vi "Documentation.vi"   [LabVIEW 2019, in "Instrument.AFM_DLog.lvclass"]
uses:
  Instrument.AFM_DLog.lvclass
  d6248588-9140-4ff5-86c8-21cd21a7458c.vi
  7f72b22a-d2f9-4e7f-a221-6a14f9895fe8.vi
  7f72b22a-d2f9-4e7f-a221-6a14f9895fe8.vi/42f86bcf-068c-4498-966d-034f8f180634.vi
  7f72b22a-d2f9-4e7f-a221-6a14f9895fe8.vi/bd09be8a-821b-4106-aeb3-ddc481226dfb.vi
  <vilib>/Utility/Data Type/Get Type Information.vi
  <vilib>/Utility/Data Type/Get Numeric Information.vi
  <userlib>/_OpenG.lib/lvdata/lvdata.llb/Unwrap VVariant__ogtk.vi
  <vilib>/JDP Science/JSONtext/JSON text to Variant.vi
  <userlib>/LevyLab/Instrument Framework/Instrument/Instrument.lvclass
  <vilib>/JKI/JKI SMO/SMO/SMO.lvclass
  Typedefs/Instrument.AFM_DLog.PublicCommands--Enum.ctl
  Typedefs/Instrument.AFM_DLog.getAll--Cluster.ctl
  Typedefs/Instrument.AFM_DLog.Configuration--Cluster.ctl
  Typedefs/Instrument.AFM_DLog.ProtectedCommands--Enum.ctl
  <vilib>/JDP Science/JSONtext/LVClass Serializer/JSONtext LVClass Serializer.lvclass
  <userlib>/LevyLab/Instrument Framework/Instrument UI/Instrument UI.lvclass
  <userlib>/LevyLab/Instrument Framework/Instrument Types/Amplifier/Instrument.Amplifier.lvclass
  <userlib>/LevyLab/Instrument Framework/Instrument Types/CBridge/Instrument.CBridge.lvclass
  <userlib>/LevyLab/Instrument Framework/Instrument Types/Cryostat/Instrument.Cryostat.lvclass
  <userlib>/LevyLab/Instrument Framework/Instrument Types/Delay Line/Instrument.DelayLine.lvclass
  <userlib>/LevyLab/Instrument Framework/Instrument Types/Lockin/Instrument.LockinAPI.lvclass
  <userlib>/LevyLab/Instrument Framework/Instrument Types/Strain/Instrument.Strain.lvclass
  <userlib>/LevyLab/Instrument Framework/Instrument Types/VNA/Instrument.VNA.lvclass
  <userlib>/LevyLab/Instrument Framework/Instrument Types/SCPI/Instrument.SCPI.lvclass
  <userlib>/LevyLab/Instrument Framework/Instrument Types/SignalGenerator/Instrument.SignalGenerator.lvclass
  <userlib>/LevyLab/Instrument Framework/Instrument Types/VSource/Instrument.VSource.lvclass
  Instrument UI.AFM_DLog/Instrument UI.AFM_DLog.UI--Cluster.ctl
  <vilib>/JKI/JKI SMO/SMO.UI/SMO.UI.lvclass
  C:/Program Files (x86)/National Instruments/LabVIEW 2019/user.lib/LevyLab/Instrument Framework/Instrument/Instrument.lvclass
  C:/Program Files (x86)/National Instruments/LabVIEW 2019/vi.lib/JKI/JKI SMO/SMO/SMO.lvclass
  <userlib>/LevyLab/Instrument Framework/Instrument/Typedefs/Instrument.ProtectedCommands--Enum.ctl
  <userlib>/LevyLab/Instrument Framework/Instrument/Typedefs/Instrument.Commands--Enum.ctl
types:
  T1 = typedef "Instrument.AFM_DLog.lvclass/Instrument.AFM_DLog.Configuration--Cluster.ctl" = cluster{"Example Setting 1":dbl, "Example Setting 2":dbl, "Example Setting 3":string}
  T2 = typedef "Instrument.AFM_DLog.lvclass/Instrument.AFM_DLog.getAll--Cluster.ctl" = cluster{"Name":string, "X":dbl, "Y":dbl, "Speed":dbl, "Voltage":dbl, "Set Resistance":string, "Move Setpoint":dbl, "Amplifier":dbl, "Writing Setpoint":dbl, "Interpolation":dbl}
  T3 = typedef "Instrument.AFM_DLog.lvclass/Instrument.AFM_DLog.ProtectedCommands--Enum.ctl" = enum16{"doProtected"}
  T4 = typedef "Instrument.AFM_DLog.lvclass/Instrument.AFM_DLog.PublicCommands--Enum.ctl" = enum16{"doSomething"}
  T5 = typedef "Instrument.lvlib/Instrument.lvclass/Instrument.Commands--Enum.ctl" = enum16{"ACK", "HELP", "IDN", "getAll", "getAllData"}
  T6 = typedef "Instrument.lvlib/Instrument.lvclass/Instrument.ProtectedCommands--Enum.ctl" = enum16{"setConfiguration", "setIDN", "setAll", "setAllData"}
  T7 = typedef "Instrument UI.AFM_DLog.lvclass/Instrument UI.AFM_DLog.UI--Cluster.ctl" = cluster{"Parameter":dbl, "Parameter 2":string}
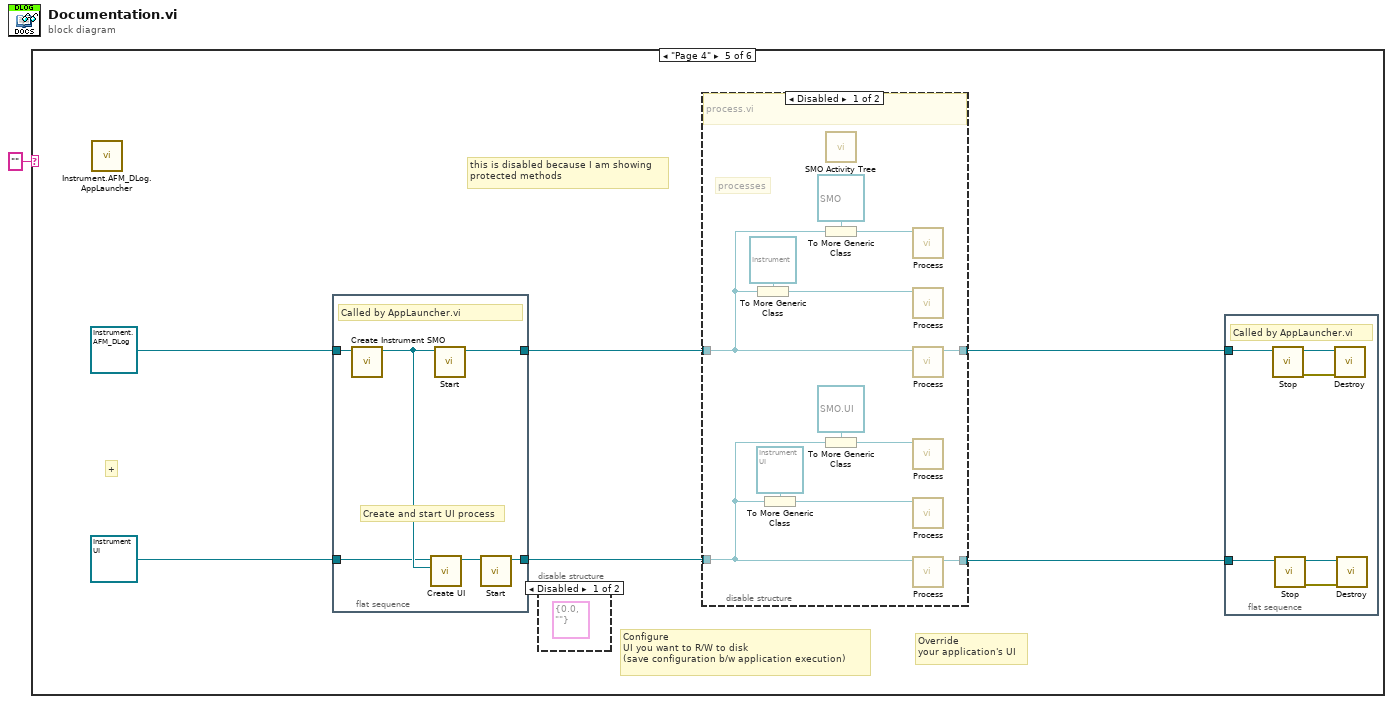
[diagram p0: block diagram]
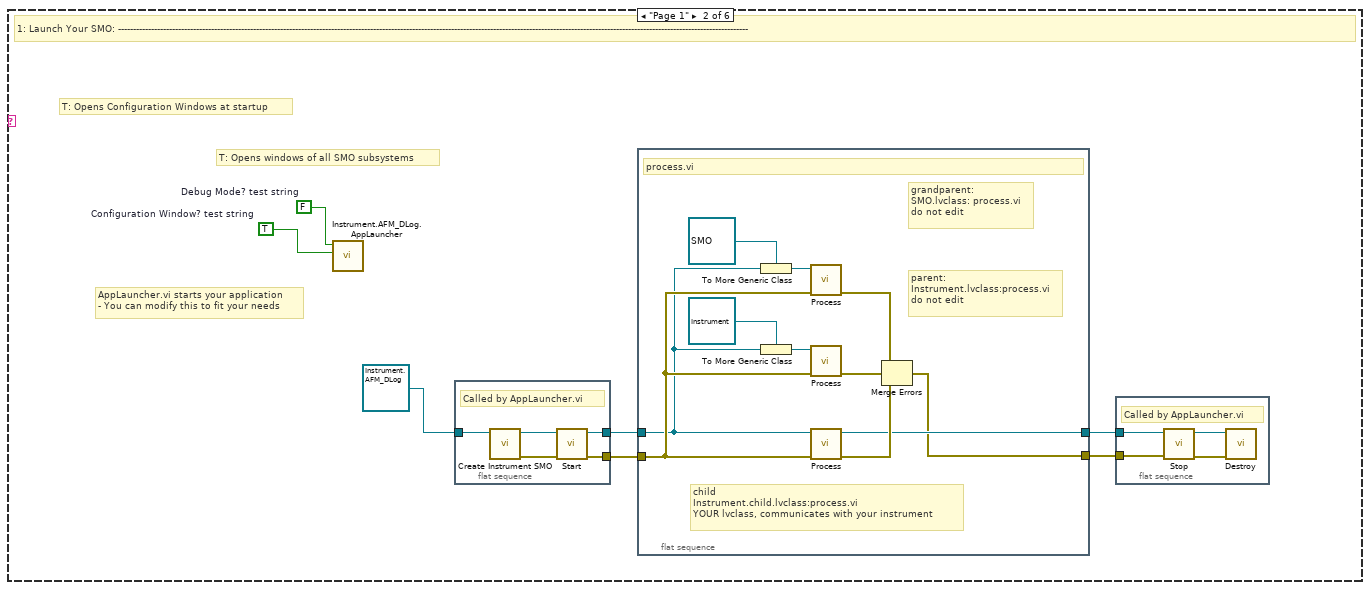
[diagram p3: hidden frame]
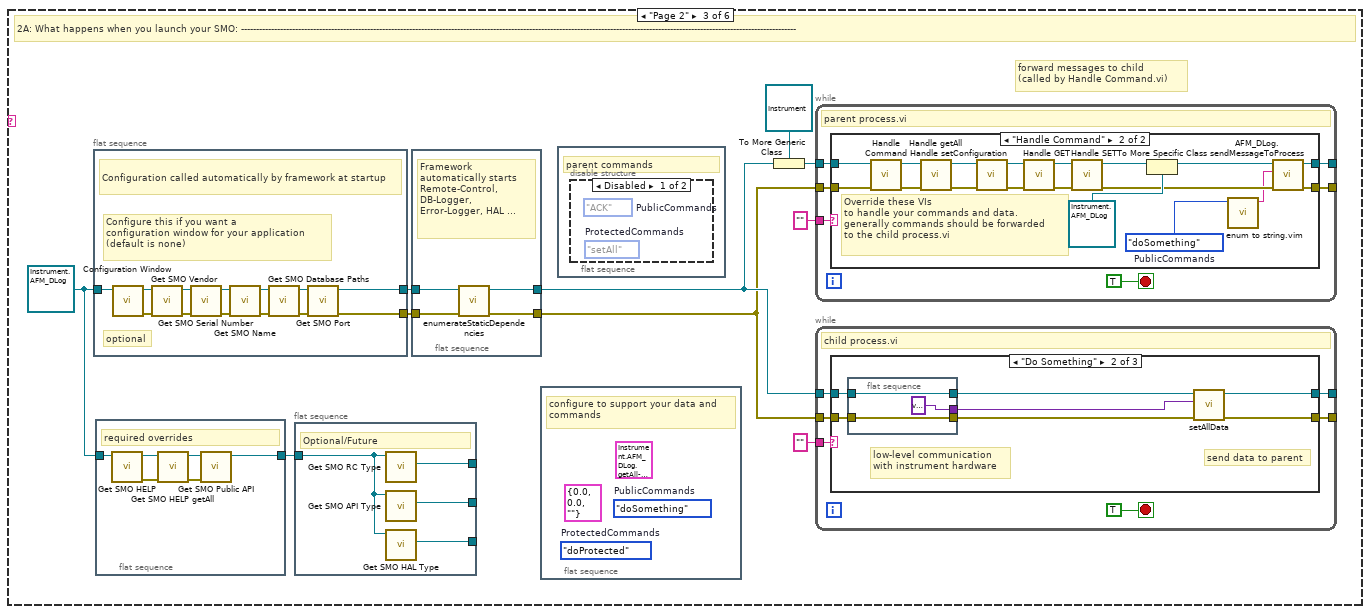
[diagram p4: hidden frame]
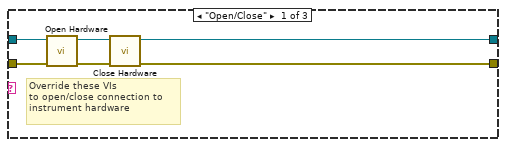
[diagram p6: hidden frame]
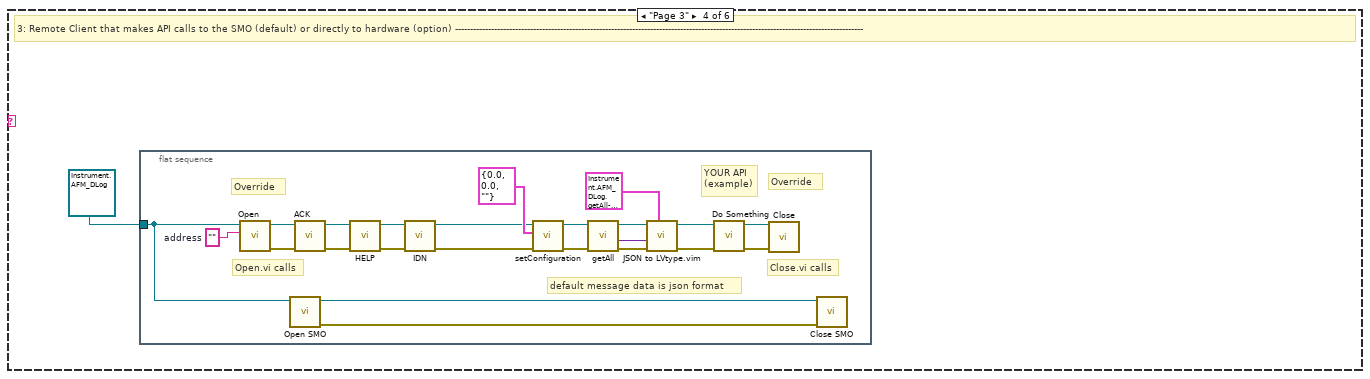
[diagram p9: hidden frame]
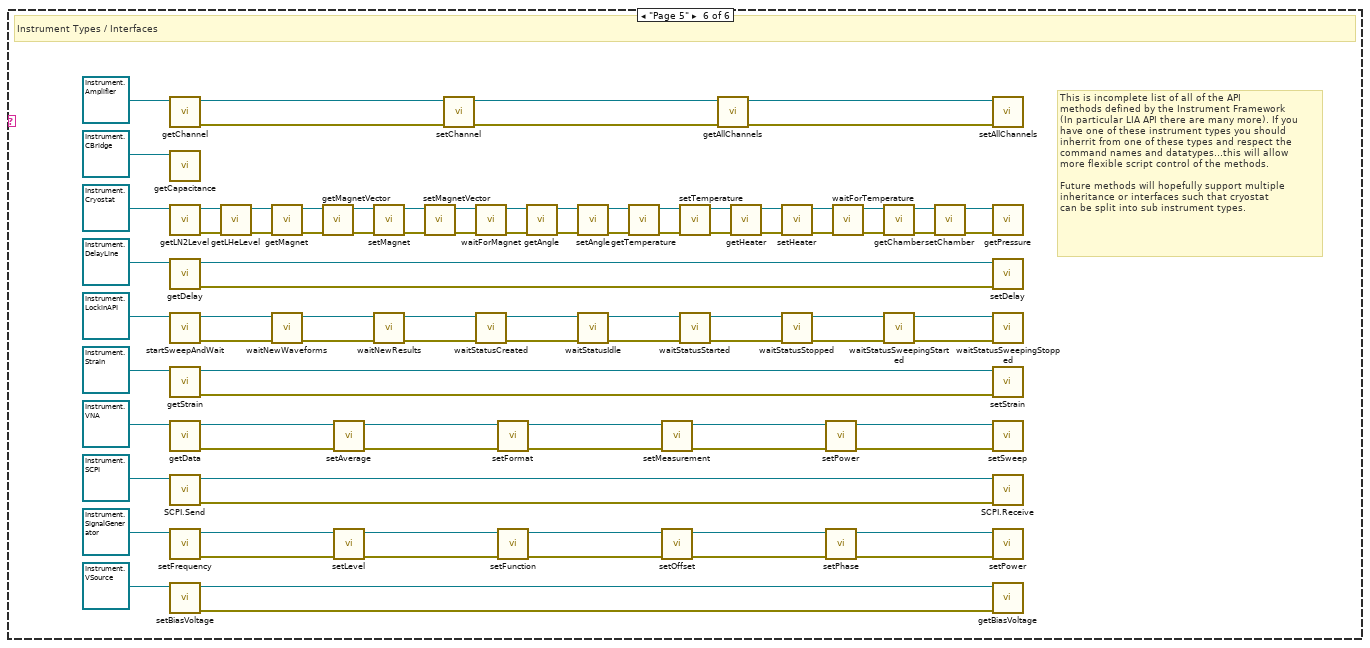
[diagram p12: hidden frame]
diagram:
  n1 = case shown="\"Page 4\"" "" {
    frame Default {
    }
    frame "Page 1" {
      w7 = TRUE  # Configuration Window? test string
      w8 = FALSE  # Debug Mode? test string
      # "AppLauncher.vi starts your application\n- You can modify this to fit your needs"
      # "T: Opens windows of all SMO subsystems"
      # "T: Opens Configuration Windows at startup"
      # "1: Launch Your SMO: ------------------------------------------------------------------------------------------------------------------------------------------------------------------------------------------------------------------"
      n2 = call "Instrument.AFM_DLog.AppLauncher.vi"("Config Window"=w7, "Debug Mode"=w8) -> ()  [unwired: 9 in, 1 out]
      n3 = flat-sequence {
        tunnel: [w26] -> w3
        tunnel: [w25] -> w5
        tunnel: refnum<class "Instrument.AFM_DLog.lvclass"> refnum ("Instrument.Template.lvclass") -> [w24]
        frame #0 {
          # "Called by AppLauncher.vi"
          n4 = call <userlib>:"Create Instrument SMO.vi"("Instrument in"=w24) -> ("error out"=w27:errorcluster, "Instrument out"=w28:refnum<class "Instrument.AFM_DLog.lvclass">)  [unwired: 9 in]
          n5 = call <vilib>:"Start.vi"("error in (no error)"=w27, "SMO"=w28) -> ("error out"=w25:errorcluster, "SMO out"=w26:refnum<class "Instrument.AFM_DLog.lvclass">)  [unwired: 8 in]
        }
      }
      n6 = flat-sequence {
        tunnel: [w10] -> w6
        tunnel: w5 -> [w18]
        tunnel: [w13] -> w4
        tunnel: w3 -> [w12]
        frame #0 {
          # "child\nInstrument.child.lvclass:process.vi\nYOUR lvclass, communicates with your instrument"
          # "grandparent:\nSMO.lvclass: process.vi\ndo not edit"
          # "parent:\nInstrument.lvclass:process.vi\ndo not edit"
          # "process.vi"
          n7 = To More Generic Class(target class=refnum<class "SMO.lvclass"> refnum ("SMO"), reference=w12) -> (generic class reference=w19:refnum<class "SMO.lvclass">)
          n8 = To More Generic Class(target class=refnum<class "Instrument.lvclass"> refnum ("Instrument"), reference=w12) -> (generic class reference=w17:refnum<class "Instrument.lvclass">)
          n9 = call-dynamic "Process.vi"("error in"=w18, "SMO"=w19) -> ("error out"=w14:errorcluster)  [unwired: 8 in, 1 out]
          n10 = call-dynamic "Process.vi"("error in"=w18, "Instrument"=w17) -> ("error out"=w16:errorcluster)  [unwired: 8 in, 1 out]
          n11 = call-dynamic "Process.vi"("error in"=w18, "Instrument.AFM_DLog in"=w12) -> ("error out"=w15:errorcluster, "Instrument.AFM_DLog out"=w13:refnum<class "Instrument.AFM_DLog.lvclass">)  [unwired: 8 in]
          n12 = Merge Errors(w14, w16, w15) -> (w10:errorcluster)
        }
      }
      n13 = flat-sequence {
        tunnel: w4 -> [w21]
        tunnel: w6 -> [w20]
        frame #0 {
          # "Called by AppLauncher.vi"
          n14 = call <vilib>:"Stop.vi"("error in (no error)"=w20, "SMO"=w21) -> ("error out"=w23:errorcluster, "SMO out"=w22:refnum<class "Instrument.AFM_DLog.lvclass">)  [unwired: 8 in]
          n15 = call <vilib>:"Destroy.vi"("error in (no error)"=w23, "SMO"=w22) -> ()  [unwired: 9 in, 1 out]
        }
      }
    }
    frame "Page 2" {
      w32 = refnum<class "Instrument.AFM_DLog.lvclass"> refnum ("Instrument.Template.lvclass")
      # "forward messages to child\n(called by Handle Command.vi)"
      # "2A: What happens when you launch your SMO: -----------------------------------------------------------------------------------------------------------------------------------------------------------------------------------------"
      n16 = flat-sequence {
        tunnel: w32 -> [w59]
        tunnel: [w49] -> w33
        tunnel: [w50] -> w34
        frame #0 {
          # "optional"
          # "Configure this if you want a\nconfiguration window for your application\n(default is none)"
          # "Configuration called automatically by framework at startup"
          n17 = call-dynamic "Configuration Window.vi"("Example Instrument in"=w59) -> ("error out"=w61:errorcluster, "Example Instrument out"=w60:refnum<class "Instrument.AFM_DLog.lvclass">)  [unwired: 9 in]
          n18 = call-dynamic "Get SMO Vendor.vi"("error in (no error)"=w61, "Instrument.AFM_DLog in"=w60) -> ("error out"=w51:errorcluster, "Instrument.AFM_DLog out"=w56:refnum<class "Instrument.AFM_DLog.lvclass">)  [unwired: 7 in, 1 out]
          n19 = call-dynamic "Get SMO Serial Number.vi"("error in (no error)"=w51, "Instrument.AFM_DLog in"=w56) -> ("error out"=w52:errorcluster, "Instrument.AFM_DLog out"=w55:refnum<class "Instrument.AFM_DLog.lvclass">)  [unwired: 7 in, 1 out]
          n20 = call-dynamic "Get SMO Name.vi"("error in (no error)"=w52, "Instrument.AFM_DLog in"=w55) -> ("error out"=w53:errorcluster, "Instrument.AFM_DLog out"=w54:refnum<class "Instrument.AFM_DLog.lvclass">)  [unwired: 7 in, 1 out]
          n21 = call-dynamic "Get SMO Database Paths.vi"("error in (no error)"=w53, "Instrument.AFM_DLog in"=w54) -> ("error out"=w57:errorcluster, "Instrument.AFM_DLog out"=w58:refnum<class "Instrument.AFM_DLog.lvclass">)  [unwired: 7 in, 1 out]
          n22 = call-dynamic "Get SMO Port.vi"("error in (no error)"=w57, "Instrument.AFM_DLog in"=w58) -> ("error out"=w49:errorcluster, "Instrument.AFM_DLog out"=w50:refnum<class "Instrument.AFM_DLog.lvclass">)  [unwired: 7 in, 1 out]
        }
      }
      n23 = flat-sequence {
        tunnel: w32 -> [w40]
        tunnel: [w39] -> w31
        frame #0 {
          # "required overrides"
          n24 = call-dynamic "Get SMO HELP.vi"("Instrument.AFM_DLog in"=w40) -> ("error out"=w44:errorcluster, "Instrument.AFM_DLog out"=w43:refnum<class "Instrument.AFM_DLog.lvclass">)  [unwired: 8 in, 1 out]
          n25 = call-dynamic "Get SMO HELP getAll.vi"("error in (no error)"=w44, "Instrument.AFM_DLog in"=w43) -> ("error out"=w41:errorcluster, "Instrument.AFM_DLog out"=w42:refnum<class "Instrument.AFM_DLog.lvclass">)  [unwired: 7 in, 1 out]
          n26 = call-dynamic "Get SMO Public API.vi"("error in (no error)"=w41, "Instrument.AFM_DLog in"=w42) -> ("Instrument.AFM_DLog out"=w39:refnum<class "Instrument.AFM_DLog.lvclass">)  [unwired: 7 in, 2 out]
        }
      }
      n27 = flat-sequence {
        tunnel: w31 -> [w65]
        tunnel: [w64] -> _
        tunnel: [w63] -> _
        tunnel: [w62] -> _
        frame #0 {
          # "Optional/Future"
          n28 = call-dynamic "Get SMO RC Type.vi"("Instrument in"=w65) -> ("RemoteControl"=w64:refnum<class "RemoteControl.lvclass">)  [unwired: 8 in, 2 out]
          n29 = call-dynamic "Get SMO API Type.vi"("Instrument in"=w65) -> ("API"=w63:refnum<class "API.lvclass">)  [unwired: 8 in, 2 out]
          n30 = call-dynamic "Get SMO HAL Type.vi"("Instrument in"=w65) -> ("Dependencies.HAL"=w62:refnum<class "HAL.lvclass">)  [unwired: 8 in, 2 out]
        }
      }
      n31 = flat-sequence {
        tunnel: w34 -> [w48]
        tunnel: w33 -> [w47]
        tunnel: [w46] -> w30
        tunnel: [w45] -> w29
        frame #0 {
          # "Framework automatically starts\nRemote-Control, DB-Logger, Error-Logger, HAL ..."
          n32 = call-dynamic "enumerateStaticDependencies.vi"("error in (no error)"=w47, "Instrument"=w48) -> ("error out"=w45:errorcluster, "Instrument out"=w46:refnum<class "Instrument.AFM_DLog.lvclass">)  [unwired: 7 in, 1 out]
        }
      }
      n33 = flat-sequence {
        frame #0 {
          (unwired) Instrument.AFM_DLog.ProtectedCommands--Enum."doProtected"  # ProtectedCommands
          (unwired) T1 {"Example Setting 1"=0.0, "Example Setting 2"=0.0, "Example Setting 3"=""} ("Configuration")
          (unwired) T2 {"Name"="", "X"=0.0, "Y"=0.0, "Speed"=0.0, "Voltage"=0.0, "Set Resistance"="", "Move Setpoint"=0.0, "Amplifier"=0.0, "Writing Setpoint"=0.0, "Interpolation"=0.0} ("getAll")
          (unwired) Instrument.AFM_DLog.PublicCommands--Enum."doSomething"  # PublicCommands
          # "configure to support your data and commands"
        }
      }
      n34 = flat-sequence {
        frame #0 {
          # "parent commands"
          n35 = disable-structure shown="Disabled" {
            frame Disabled {
              (unwired) Instrument.Commands--Enum."ACK"  # PublicCommands
              (unwired) Instrument.ProtectedCommands--Enum."setAll"  # ProtectedCommands
            }
            frame Enabled {
            }
          }
        }
      }
      n36 = To More Generic Class(target class=refnum<class "Instrument.lvclass"> refnum ("Instrument"), reference=w30) -> (generic class reference=w35:refnum<class "Instrument.lvclass">)
      n37 = while {
        tunnel: "" -> [w95]
        tunnel: w35 -> [w93]
        tunnel: [w92] -> _
        tunnel: w29 -> [w91]
        tunnel: [w90] -> _
        stop <- TRUE stop-if-true
        # "parent process.vi"
        n38 = case shown="\"Handle Command\"" w95 {
          tunnel: w93 -> [w97 w115]
          tunnel: [w97 w109] -> w92
          tunnel: w91 -> [w96 w114]
          tunnel: [w96 w108] -> w90
          frame Default {
          }
          frame "Handle Command" {
            w99 = Instrument.AFM_DLog.PublicCommands--Enum."doSomething"  # PublicCommands
            # "Override these VIs\nto handle your commands and data.\ngenerally commands should be forwarded\nto the child process.vi"
            n39 = call-dynamic "Handle Command.vi"("error in (no error)"=w114, "Instrument in"=w115) -> ("error out"=w110:errorcluster, "Instrument out"=w113:refnum<class "Instrument.lvclass">)  [unwired: 6 in, 2 out]
            n40 = call-dynamic "Handle getAll.vi"("error in (no error)"=w110, "Instrument in"=w113) -> ("error out"=w111:errorcluster, "Instrument out"=w112:refnum<class "Instrument.lvclass">)  [unwired: 7 in, 1 out]
            n41 = call-dynamic "Handle setConfiguration.vi"("error in (no error)"=w111, "Instrument in"=w112) -> ("error out"=w104:errorcluster, "Instrument out"=w105:refnum<class "Instrument.lvclass">)  [unwired: 8 in]
            n42 = call-dynamic "Handle GET.vi"("error in (no error)"=w104, "Instrument in"=w105) -> ("error out"=w102:errorcluster, "Instrument out"=w103:refnum<class "Instrument.lvclass">)  [unwired: 7 in, 1 out]
            n43 = call-dynamic "Handle SET.vi"("error in (no error)"=w102, "Instrument in"=w103) -> ("error out"=w100:errorcluster, "Instrument out"=w101:refnum<class "Instrument.lvclass">)  [unwired: 7 in, 1 out]
            n44 = To More Specific Class(target class=refnum<class "Instrument.AFM_DLog.lvclass"> refnum ("Instrument.Template.lvclass"), reference=w101) -> (specific class reference=w107:refnum<class "Instrument.AFM_DLog.lvclass">)  [unwired: 1 in, 1 out]
            n45 = call "enum to string.vim"("enum in"=w99) -> ("string out"=w98:string)  [unwired: 9 in, 1 out]
            n46 = call "AFM_DLog.sendMessageToProcess.vi"("error in (no error)"=w100, "Command"=w98, "Instrument.AFM_DLog in"=w107) -> ("error out"=w108:errorcluster, "Instrument.AFM_DLog out"=w109:refnum<class "Instrument.AFM_DLog.lvclass">)  [unwired: 7 in]
          }
        }
      }
      n47 = while {
        tunnel: "" -> [w71]
        tunnel: w30 -> [w69]
        tunnel: [w68] -> _
        tunnel: w29 -> [w67]
        tunnel: [w66] -> _
        stop <- TRUE stop-if-true
        # "child process.vi"
        n48 = case shown="\"Do Something\"" w71 {
          tunnel: w69 -> [w74 w83 w89]
          tunnel: [w73 w80 w89] -> w68
          tunnel: w67 -> [w77 w84 w88]
          tunnel: [w72 w79 w88] -> w66
          frame "Open/Close" {
            # "Override these VIs\nto open/close connection to\ninstrument hardware"
            n49 = call-dynamic "Open Hardware.vi"("error in (no error)"=w77, "Instrument in"=w74) -> ("error out"=w76:errorcluster, "Instrument out"=w75:refnum<class "Instrument.AFM_DLog.lvclass">)  [unwired: 8 in]
            n50 = call-dynamic "Close Hardware.vi"("error in (no error)"=w76, "Instrument in"=w75) -> ("error out"=w72:errorcluster, "Instrument out"=w73:refnum<class "Instrument.AFM_DLog.lvclass">)  [unwired: 8 in]
          }
          frame "Do Something" {
            # "low-level communication\nwith instrument hardware"
            # "send data to parent"
            n51 = flat-sequence {
              tunnel: w84 -> [w87]
              tunnel: [w87] -> w78
              tunnel: w83 -> [w86]
              tunnel: [w86] -> w81
              tunnel: [variant ("Data")] -> w82
              frame #0 {
              }
            }
            n52 = call <userlib>:"setAllData.vi"("error in (no error)"=w78, "AllData"=w82, "Instrument in"=w81) -> ("error out"=w79:errorcluster, "Instrument out"=w80:refnum<class "Instrument.AFM_DLog.lvclass">)  [unwired: 7 in]
          }
          frame Default {
          }
        }
      }
    }
    frame "Page 3" {
      # "3: Remote Client that makes API calls to the SMO (default) or directly to hardware (option) ----------------------------------------------------------------------------------------------------------------------------------------"
      n53 = flat-sequence {
        tunnel: refnum<class "Instrument.AFM_DLog.lvclass"> refnum ("Instrument.Template.lvclass") -> [w126]
        frame #0 {
          w129 = ""  # address
          # "default message data is json format"
          # "Close.vi calls"
          # "Open.vi calls"
          # "YOUR API\n(example)"
          # "Override"
          # "Override"
          n54 = call-dynamic "Open.vi"("address"=w129, "Instrument.AFM_DLog in"=w126) -> ("error out"=w138:errorcluster, "Instrument.AFM_DLog out"=w137:refnum<class "Instrument.AFM_DLog.lvclass">)  [unwired: 8 in]
          n55 = call <userlib>:"Open SMO.vi"("Instrument in"=w126) -> ("error out"=w127:errorcluster, "Instrument out"=w128:refnum<class "Instrument.AFM_DLog.lvclass">)  [unwired: 9 in]
          n56 = call <userlib>:"ACK.vi"("error in (no error)"=w138, "Instrument in"=w137) -> ("error out"=w136:errorcluster, "Instrument out"=w135:refnum<class "Instrument.AFM_DLog.lvclass">)  [unwired: 7 in, 1 out]
          n57 = call <userlib>:"HELP.vi"("error in (no error)"=w136, "Instrument in"=w135) -> ("error out"=w119:errorcluster, "Instrument in"=w120:refnum<class "Instrument.AFM_DLog.lvclass">)  [unwired: 7 in, 1 out]
          n58 = call <userlib>:"IDN.vi"("error in (no error)"=w119, "Instrument in"=w120) -> ("error out"=w117:errorcluster, "Instrument in"=w118:refnum<class "Instrument.AFM_DLog.lvclass">)  [unwired: 7 in, 1 out]
          n59 = call <userlib>:"setConfiguration.vi"("error in (no error)"=w117, "Configuration"=T1 {"Example Setting 1"=0.0, "Example Setting 2"=0.0, "Example Setting 3"=""}, "Instrument in"=w118) -> ("error out"=w130:errorcluster, "Instrument out"=w131:refnum<class "Instrument.AFM_DLog.lvclass">)  [unwired: 7 in]
          n60 = call <userlib>:"getAll.vi"("error in (no error)"=w130, "Instrument in"=w131) -> ("error out"=w125:errorcluster, "getAll"=w121:variant, "Instrument out"=w122:refnum<class "Instrument.AFM_DLog.lvclass">)  [unwired: 7 in]
          n61 = call "JSON to LVtype.vim"("type"=T2 {"Name"="", "X"=0.0, "Y"=0.0, "Speed"=0.0, "Voltage"=0.0, "Set Resistance"="", "Move Setpoint"=0.0, "Amplifier"=0.0, "Writing Setpoint"=0.0, "Interpolation"=0.0} ("getAll"), "error in (no error)"=w125, "JSON Data in"=w121) -> ("error out"=w123:errorcluster)  [unwired: 7 in, 1 out]
          n62 = call-dynamic "Do Something.vi"("error in (no error)"=w123, "Instrument.AFM_DLog in"=w122) -> ("error out"=w133:errorcluster, "Instrument.AFM_DLog out"=w134:refnum<class "Instrument.AFM_DLog.lvclass">)  [unwired: 8 in]
          n63 = call-dynamic "Close.vi"("error in (no error)"=w133, "Instrument.AFM_DLog in"=w134) -> ()  [unwired: 8 in, 2 out]
          n64 = call <userlib>:"Close SMO.vi"("error in (no error)"=w127, "Instrument in"=w128) -> ()  [unwired: 8 in, 2 out]
        }
      }
    }
    frame "Page 4" {
      # "this is disabled because I am showing\nprotected methods"
      # "Configure\nUI you want to R/W to disk\n(save configuration b/w application execution)"
      # "Override\nyour application's UI"
      # "+"
      n65 = call "Instrument.AFM_DLog.AppLauncher.vi"() -> ()  [unwired: 11 in, 1 out]
      n66 = flat-sequence {
        tunnel: [w156] -> w142
        tunnel: refnum<class "Instrument.AFM_DLog.lvclass"> refnum ("Instrument.Template.lvclass") -> [w155]
        tunnel: refnum<class "Instrument UI.lvclass"> refnum ("Instrument UI.Template.lvclass") -> [w153]
        tunnel: [w151] -> w140
        frame #0 {
          # "Create and start UI process"
          # "Called by AppLauncher.vi"
          n67 = call <userlib>:"Create Instrument SMO.vi"("Instrument in"=w155) -> ("Instrument out"=w154:refnum<class "Instrument.AFM_DLog.lvclass">)  [unwired: 9 in, 1 out]
          n68 = call <userlib>:"Create UI.vi"("Instrument in"=w154, "Instrument UI"=w153) -> ("Instrument UI out"=w152:refnum<class "Instrument UI.lvclass">)  [unwired: 8 in, 1 out]
          n69 = call <vilib>:"Start.vi"("SMO"=w154) -> ("SMO out"=w156:refnum<class "Instrument.AFM_DLog.lvclass">)  [unwired: 9 in, 1 out]
          n70 = call <vilib>:"Start.vi"("SMO"=w152) -> ("SMO out"=w151:refnum<class "Instrument UI.lvclass">)  [unwired: 9 in, 1 out]
        }
      }
      n71 = disable-structure shown="Disabled" {
        frame Disabled {
          (unwired) T7 {"Parameter"=0.0, "Parameter 2"=""} ("UI")
        }
        frame Enabled {
        }
      }
      n72 = disable-structure shown="Disabled" {
        disable-tunnel: [w168 w170] -> w143
        disable-tunnel: w142 -> [w167 w170]
        disable-tunnel: w140 -> [w166 w169]
        disable-tunnel: [w165 w169] -> w139
        frame Disabled {
          # "processes"
          # "process.vi"
          n73 = To More Generic Class(target class=refnum<class "Instrument.lvclass"> refnum ("Instrument"), reference=w167) -> (generic class reference=w163:refnum<class "Instrument.lvclass">)
          n74 = To More Generic Class(target class=refnum<class "Instrument UI.lvclass"> refnum ("Instrument UI"), reference=w166) -> (generic class reference=w159:refnum<class "Instrument UI.lvclass">)
          n75 = call <vilib>:"SMO Activity Tree.vi"() -> ()  [unwired: 12 in]
          n76 = To More Generic Class(target class=refnum<class "SMO.lvclass"> refnum ("SMO"), reference=w167) -> (generic class reference=w164:refnum<class "SMO.lvclass">)
          n77 = To More Generic Class(target class=refnum<class "SMO.UI.lvclass"> refnum ("SMO.UI"), reference=w166) -> (generic class reference=w157:refnum<class "SMO.UI.lvclass">)
          n78 = call-dynamic "Process.vi"("SMO"=w164) -> ()  [unwired: 9 in, 2 out]
          n79 = call-dynamic "Process.vi"("Instrument"=w163) -> ()  [unwired: 9 in, 2 out]
          n80 = call-dynamic "Process.vi"("Instrument.AFM_DLog in"=w167) -> ("Instrument.AFM_DLog out"=w168:refnum<class "Instrument.AFM_DLog.lvclass">)  [unwired: 9 in, 1 out]
          n81 = call-dynamic "Process.vi"("SMO.UI"=w157) -> ()  [unwired: 9 in, 2 out]
          n82 = call-dynamic "Process.vi"("Instrument UI in"=w159) -> ()  [unwired: 9 in, 2 out]
          n83 = call-dynamic "Process.vi"("Instrument UI in"=w166) -> ("Instrument UI out"=w165:refnum<class "Instrument UI.lvclass">)  [unwired: 9 in, 1 out]
        }
        frame Enabled {
        }
      }
      n84 = flat-sequence {
        tunnel: w143 -> [w148]
        tunnel: w139 -> [w146]
        frame #0 {
          # "Called by AppLauncher.vi"
          n85 = call <vilib>:"Stop.vi"("SMO"=w148) -> ("error out"=w150:errorcluster, "SMO out"=w149:refnum<class "Instrument.AFM_DLog.lvclass">)  [unwired: 9 in]
          n86 = call <vilib>:"Stop.vi"("SMO"=w146) -> ("error out"=w147:errorcluster, "SMO out"=w145:refnum<class "Instrument UI.lvclass">)  [unwired: 9 in]
          n87 = call <vilib>:"Destroy.vi"("error in (no error)"=w150, "SMO"=w149) -> ()  [unwired: 9 in, 1 out]
          n88 = call <vilib>:"Destroy.vi"("error in (no error)"=w147, "SMO"=w145) -> ()  [unwired: 9 in, 1 out]
        }
      }
    }
    frame "Page 5" {
      # "This is incomplete list of all of the API\nmethods defined by the Instrument Framework\n(In particular LIA API there are many more). If you\nhave one of these instrument types you should\ninherrit from one of these types and respect the \ncommand names and datatypes...this will allow\nmore flexible script control of the methods.\n\nFuture methods will hopefully support multiple\ninheritance or interfaces such that cryostat\ncan be split into sub instrument types."
      # "Instrument Types / Interfaces"
      n89 = call-dynamic "getChannel.vi"("Instrument.Amplifier in"=refnum<class "Instrument.Amplifier.lvclass"> refnum ("Instrument.Amplifier.lvclass")) -> ("error out"=w251:errorcluster, "Instrument.Amplifier out"=w252:refnum<class "Instrument.Amplifier.lvclass">)  [unwired: 8 in, 1 out]
      n90 = call-dynamic "getCapacitance.vi"("Instrument.CBridge in"=refnum<class "Instrument.CBridge.lvclass"> refnum ("Instrument.CBridge.lvclass")) -> ()  [unwired: 8 in, 3 out]
      n91 = call-dynamic "getLN2Level.vi"("Instrument.Cryostat in"=refnum<class "Instrument.Cryostat.lvclass"> refnum ("Instrument.Cryostat.lvclass")) -> ("error out"=w245:errorcluster, "Instrument.Cryostat out"=w246:refnum<class "Instrument.Cryostat.lvclass">)  [unwired: 8 in, 1 out]
      n92 = call <userlib>:"getDelay.vi"("Instrument.DelayLine in"=refnum<class "Instrument.DelayLine.lvclass"> refnum ("Instrument.DelayLine.lvclass")) -> ("error out"=w213:errorcluster, "Instrument.DelayLine out"=w214:refnum<class "Instrument.DelayLine.lvclass">)  [unwired: 7 in, 2 out]
      n93 = call-dynamic "startSweepAndWait.vi"("Instrument.LockinAPI in"=refnum<class "Instrument.LockinAPI.lvclass"> refnum ("Instrument.LockinAPI.lvclass")) -> ("error out"=w211:errorcluster, "Instrument.LockinAPI out"=w212:refnum<class "Instrument.LockinAPI.lvclass">)  [unwired: 9 in]
      n94 = call-dynamic "getStrain.vi"("Instrument.Strain in"=refnum<class "Instrument.Strain.lvclass"> refnum ("Instrument.Strain.lvclass")) -> ("error out"=w195:errorcluster, "Instrument.Strain out"=w196:refnum<class "Instrument.Strain.lvclass">)  [unwired: 8 in, 1 out]
      n95 = call-dynamic "getData.vi"("Instrument.VSource in"=refnum<class "Instrument.VNA.lvclass"> refnum ("Instrument.VNA.lvclass")) -> ("error out"=w193:errorcluster, "Instrument.VSource out"=w194:refnum<class "Instrument.VNA.lvclass">)  [unwired: 8 in, 1 out]
      n96 = call-dynamic "SCPI.Send.vi"("Instrument.SCPI in"=refnum<class "Instrument.SCPI.lvclass"> refnum ("Instrument.SCPI.lvclass")) -> ("error out"=w183:errorcluster, "Instrument.SCPI out"=w184:refnum<class "Instrument.SCPI.lvclass">)  [unwired: 9 in]
      n97 = call-dynamic "setFrequency.vi"("Instrument.SignalGenerator in"=refnum<class "Instrument.SignalGenerator.lvclass"> refnum ("Instrument.SignalGenerator.lvclass")) -> ("error out"=w181:errorcluster, "Instrument.SignalGenerator out"=w182:refnum<class "Instrument.SignalGenerator.lvclass">)  [unwired: 9 in]
      n98 = call-dynamic "setBiasVoltage.vi"("Instrument.VSource in"=refnum<class "Instrument.VSource.lvclass"> refnum ("Instrument.VSource.lvclass")) -> ("error out"=w171:errorcluster, "Instrument.VSource out"=w172:refnum<class "Instrument.VSource.lvclass">)  [unwired: 9 in]
      n99 = call-dynamic "getLHeLevel.vi"("error in (no error)"=w245, "Instrument.Cryostat in"=w246) -> ("error out"=w243:errorcluster, "Instrument.Cryostat out"=w244:refnum<class "Instrument.Cryostat.lvclass">)  [unwired: 7 in, 1 out]
      n100 = call-dynamic "getMagnet.vi"("error in (no error)"=w243, "Instrument.Cryostat in"=w244) -> ("error out"=w241:errorcluster, "Instrument.Cryostat out"=w242:refnum<class "Instrument.Cryostat.lvclass">)  [unwired: 5 in, 3 out]
      n101 = call-dynamic "waitNewWaveforms.vi"("error in (no error)"=w211, "Instrument.LockinAPI in"=w212) -> ("error out"=w209:errorcluster, "Instrument.LockinAPI out"=w210:refnum<class "Instrument.LockinAPI.lvclass">)  [unwired: 7 in, 1 out]
      n102 = call-dynamic "getMagnetVector.vi"("error in (no error)"=w241, "Instrument.Cryostat in"=w242) -> ("error out"=w239:errorcluster, "Instrument.Cryostat out"=w240:refnum<class "Instrument.Cryostat.lvclass">)  [unwired: 5 in, 3 out]
      n103 = call-dynamic "setAverage.vi"("error in (no error)"=w193, "Instrument.VSource in"=w194) -> ("error out"=w191:errorcluster, "Instrument.VSource out"=w192:refnum<class "Instrument.VNA.lvclass">)  [unwired: 8 in]
      n104 = call-dynamic "setLevel.vi"("error in (no error)"=w181, "Instrument.SignalGenerator in"=w182) -> ("error out"=w179:errorcluster, "Instrument.SignalGenerator out"=w180:refnum<class "Instrument.SignalGenerator.lvclass">)  [unwired: 8 in]
      n105 = call-dynamic "setMagnet.vi"("error in (no error)"=w239, "Instrument.Cryostat in"=w240) -> ("error out"=w237:errorcluster, "Instrument.Cryostat out"=w238:refnum<class "Instrument.Cryostat.lvclass">)  [unwired: 8 in]
      n106 = call-dynamic "waitNewResults.vi"("error in (no error)"=w209, "Instrument.LockinAPI in"=w210) -> ("error out"=w207:errorcluster, "Instrument.LockinAPI out"=w208:refnum<class "Instrument.LockinAPI.lvclass">)  [unwired: 7 in, 1 out]
      n107 = call-dynamic "setMagnetVector.vi"("error in (no error)"=w237, "Instrument.Cryostat in"=w238) -> ("error out"=w235:errorcluster, "Instrument.Cryostat out"=w236:refnum<class "Instrument.Cryostat.lvclass">)  [unwired: 8 in]
      n108 = call-dynamic "setChannel.vi"("error in (no error)"=w251, "Instrument.Amplifier in"=w252) -> ("error out"=w249:errorcluster, "Instrument.Amplifier out"=w250:refnum<class "Instrument.Amplifier.lvclass">)  [unwired: 8 in]
      n109 = call <userlib>:"waitForMagnet.vi"("error in (no error)"=w235, "Instrument.Cryostat in"=w236) -> ("error out"=w233:errorcluster, "Instrument.Cryostat out"=w234:refnum<class "Instrument.Cryostat.lvclass">)  [unwired: 8 in]
      n110 = call-dynamic "waitStatusCreated.vi"("error in (no error)"=w207, "Instrument.LockinAPI in"=w208) -> ("error out"=w205:errorcluster, "Instrument.LockinAPI out"=w206:refnum<class "Instrument.LockinAPI.lvclass">)  [unwired: 8 in]
      n111 = call-dynamic "setFormat.vi"("error in (no error)"=w191, "Instrument.VSource in"=w192) -> ("error out"=w189:errorcluster, "Instrument.VSource out"=w190:refnum<class "Instrument.VNA.lvclass">)  [unwired: 8 in]
      n112 = call-dynamic "setFunction.vi"("error in (no error)"=w179, "Instrument.SignalGenerator in"=w180) -> ("error out"=w177:errorcluster, "Instrument.SignalGenerator out"=w178:refnum<class "Instrument.SignalGenerator.lvclass">)  [unwired: 8 in]
      n113 = call-dynamic "getAngle.vi"("error in (no error)"=w233, "Instrument.Cryostat in"=w234) -> ("error out"=w231:errorcluster, "Instrument.Cryostat out"=w232:refnum<class "Instrument.Cryostat.lvclass">)  [unwired: 5 in, 3 out]
      n114 = call-dynamic "setAngle.vi"("error in (no error)"=w231, "Instrument.Cryostat in"=w232) -> ("error out"=w229:errorcluster, "Instrument.Cryostat out"=w230:refnum<class "Instrument.Cryostat.lvclass">)  [unwired: 8 in]
      n115 = call-dynamic "waitStatusIdle.vi"("error in (no error)"=w205, "Instrument.LockinAPI in"=w206) -> ("error out"=w203:errorcluster, "Instrument.LockinAPI out"=w204:refnum<class "Instrument.LockinAPI.lvclass">)  [unwired: 8 in]
      n116 = call-dynamic "getTemperature.vi"("error in (no error)"=w229, "Instrument.Cryostat in"=w230) -> ("error out"=w227:errorcluster, "Instrument.Cryostat out"=w228:refnum<class "Instrument.Cryostat.lvclass">)  [unwired: 5 in, 3 out]
      n117 = call-dynamic "setMeasurement.vi"("error in (no error)"=w189, "Instrument.VSource in"=w190) -> ("error out"=w187:errorcluster, "Instrument.VSource out"=w188:refnum<class "Instrument.VNA.lvclass">)  [unwired: 8 in]
      n118 = call-dynamic "setOffset.vi"("error in (no error)"=w177, "Instrument.SignalGenerator in"=w178) -> ("error out"=w175:errorcluster, "Instrument.SignalGenerator out"=w176:refnum<class "Instrument.SignalGenerator.lvclass">)  [unwired: 8 in]
      n119 = call-dynamic "setTemperature.vi"("error in (no error)"=w227, "Instrument.Cryostat in"=w228) -> ("error out"=w225:errorcluster, "Instrument.Cryostat out"=w226:refnum<class "Instrument.Cryostat.lvclass">)  [unwired: 8 in]
      n120 = call-dynamic "waitStatusStarted.vi"("error in (no error)"=w203, "Instrument.LockinAPI in"=w204) -> ("error out"=w201:errorcluster, "Instrument.LockinAPI out"=w202:refnum<class "Instrument.LockinAPI.lvclass">)  [unwired: 8 in]
      n121 = call-dynamic "getAllChannels.vi"("error in (no error)"=w249, "Instrument.Amplifier in"=w250) -> ("error out"=w247:errorcluster, "Instrument.Amplifier out"=w248:refnum<class "Instrument.Amplifier.lvclass">)  [unwired: 7 in, 1 out]
      n122 = call-dynamic "getHeater.vi"("error in (no error)"=w225, "Instrument.Cryostat in"=w226) -> ("error out"=w223:errorcluster, "Instrument.Cryostat out"=w224:refnum<class "Instrument.Cryostat.lvclass">)  [unwired: 6 in, 2 out]
      n123 = call-dynamic "setHeater.vi"("error in (no error)"=w223, "Instrument.Cryostat in"=w224) -> ("error out"=w221:errorcluster, "Instrument.Cryostat out"=w222:refnum<class "Instrument.Cryostat.lvclass">)  [unwired: 8 in]
      n124 = call-dynamic "waitStatusStopped.vi"("error in (no error)"=w201, "Instrument.LockinAPI in"=w202) -> ("error out"=w199:errorcluster, "Instrument.LockinAPI out"=w200:refnum<class "Instrument.LockinAPI.lvclass">)  [unwired: 8 in]
      n125 = call-dynamic "setPower.vi"("error in (no error)"=w187, "Instrument.VSource in"=w188) -> ("error out"=w185:errorcluster, "Instrument.VSource out"=w186:refnum<class "Instrument.VNA.lvclass">)  [unwired: 8 in]
      n126 = call-dynamic "setPhase.vi"("error in (no error)"=w175, "Instrument.SignalGenerator in"=w176) -> ("error out"=w173:errorcluster, "Instrument.SignalGenerator out"=w174:refnum<class "Instrument.SignalGenerator.lvclass">)  [unwired: 8 in]
      n127 = call <userlib>:"waitForTemperature.vi"("error in (no error)"=w221, "Instrument.Cryostat in"=w222) -> ("error out"=w219:errorcluster, "Instrument.Cryostat out"=w220:refnum<class "Instrument.Cryostat.lvclass">)  [unwired: 8 in]
      n128 = call-dynamic "getChamber.vi"("error in (no error)"=w219, "Instrument.Cryostat in"=w220) -> ("error out"=w217:errorcluster, "Instrument.Cryostat out"=w218:refnum<class "Instrument.Cryostat.lvclass">)  [unwired: 7 in, 1 out]
      n129 = call-dynamic "waitStatusSweepingStarted.vi"("error in (no error)"=w199, "Instrument.LockinAPI in"=w200) -> ("error out"=w197:errorcluster, "Instrument.LockinAPI out"=w198:refnum<class "Instrument.LockinAPI.lvclass">)  [unwired: 8 in]
      n130 = call-dynamic "setChamber.vi"("error in (no error)"=w217, "Instrument.Cryostat in"=w218) -> ("error out"=w215:errorcluster, "Instrument.Cryostat out"=w216:refnum<class "Instrument.Cryostat.lvclass">)  [unwired: 8 in]
      n131 = call-dynamic "setAllChannels.vi"("error in (no error)"=w247, "Instrument.Amplifier in"=w248) -> ()  [unwired: 8 in, 2 out]
      n132 = call-dynamic "getPressure.vi"("error in (no error)"=w215, "Instrument.Cryostat in"=w216) -> ()  [unwired: 6 in, 4 out]
      n133 = call-dynamic "setDelay.vi"("error in (no error)"=w213, "Instrument.Delay in"=w214) -> ()  [unwired: 8 in, 2 out]
      n134 = call-dynamic "waitStatusSweepingStopped.vi"("error in (no error)"=w197, "Instrument.LockinAPI in"=w198) -> ()  [unwired: 8 in, 2 out]
      n135 = call-dynamic "setStrain.vi"("error in (no error)"=w195, "Instrument.Strain in"=w196) -> ()  [unwired: 8 in, 2 out]
      n136 = call-dynamic "setSweep.vi"("error in (no error)"=w185, "Instrument.VSource in"=w186) -> ()  [unwired: 8 in, 2 out]
      n137 = call-dynamic "SCPI.Receive.vi"("error in (no error)"=w183, "Instrument.SCPI in"=w184) -> ()  [unwired: 7 in, 3 out]
      n138 = call-dynamic "setPower.vi"("error in (no error)"=w173, "Instrument.SignalGenerator in"=w174) -> ()  [unwired: 8 in, 2 out]
      n139 = call-dynamic "getBiasVoltage.vi"("error in (no error)"=w171, "Instrument.VSource in"=w172) -> ()  [unwired: 7 in, 3 out]
    }
  }
